vi "Increment Data.vi"(8 "error in (no error)":errorcluster, 9 "Increments In":dbl[](array[numeric])=[-0.014471871278962644, -0.0027477897622864888, 0.03594582291831433, -0.006177356244415369, -0.000527948512754489, 0.04718526152757189], 10 "LBCB Number":T2, 11 "DAO Actions":T1) -> (0 "error out":errorcluster, 1 "Increments Out":dbl[](array[numeric])=[-0.014471871278962644, -0.0027477897622864888, 0.03594582291831433, -0.006177356244415369, -0.000527948512754489, 0.04718526152757189])   [LabVIEW 2009]
uses:
  Data Access Objects/Metadata/LBCB Number.ctl
  Data Access Objects/Metadata/DAO Actions.ctl
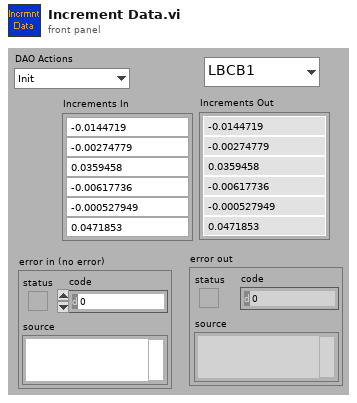
[diagram p1: front panel]
types:
  T1 = typedef "DAO Actions.ctl" = enum16{"Init", "Get", "Set"}
  T2 = typedef "LBCB Number.ctl" = enum16{"LBCB1", "LBCB2"}
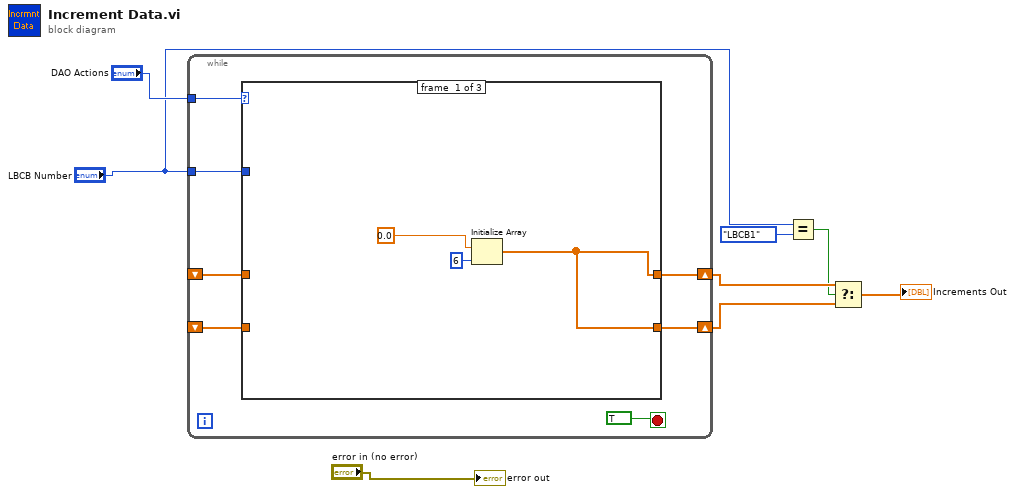
[diagram p0: block diagram]
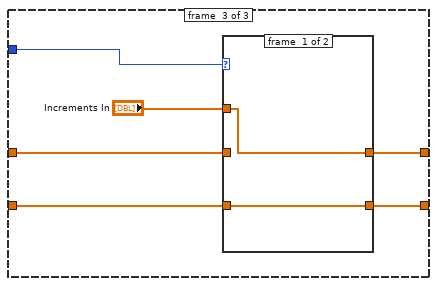
[diagram p3: hidden frame]
diagram:
  n1 = while {
    tunnel: "DAO Actions" -> [w15]
    tunnel: "LBCB Number" -> [w14]
    shift-right: [w13] -> w7
    shift-left: _ -> [w11]
    shift-right: [w12] -> w6
    shift-left: _ -> [w10]
    stop <- TRUE stop-if-true
    n2 = case shown="\"Get\"" w15 {
      tunnel: w14 -> [_ _ w26]
      tunnel: [w16 w20 w24] -> w13
      tunnel: [w16 w19 w23] -> w12
      tunnel: w11 -> [_ w20 w22]
      tunnel: w10 -> [_ w19 w21]
      frame #0 {
        n3 = Initialize Array(0.0, 6 ("dimension size")) -> (w16:dbl[])
      }
      frame #1 {
      }
      frame #2 {
        n4 = case shown="\"LBCB1\"" w26 {
          tunnel: "Increments In" -> [w28 w30]
          tunnel: [w28 w29] -> w24
          tunnel: [w27 w30] -> w23
          tunnel: w22 -> [_ w29]
          tunnel: w21 -> [w27 _]
          frame #0 {
          }
          frame #1 {
          }
        }
      }
    }
  }
  n5 = Equal?(x="LBCB Number", y=LBCB_Number."LBCB1") -> (x = y?=w1:bool)
  n6 = Select(t=w7, s=w1, f=w6) -> (s? t:f=→"Increments Out":dbl[])
  "error out" <- "error in (no error)"
